vi "test Verify with Regex Scrubber.vi"(8 "error in":errorcluster, 11 "Test Case In":refnum<class "LUnit Extensions Tests.lvclass">) -> (0 "error out":errorcluster, 3 "Test Case Out":refnum<class "LUnit Extensions Tests.lvclass">)   [LabVIEW 2020, in "LUnit Extensions Tests.lvclass"]
uses:
  LUnit Extensions Tests.lvclass
  C:/Program Files/National Instruments/LabVIEW 2020/vi.lib/Astemes/LUnit/Test Case.lvclass
  Source/Approval Tests/Regex Scrubber/Regex Scrubber.lvclass
  <vilib>/Astemes/LUnit/Test Case.lvclass/Test Case.ctl
  240f995d-3744-484a-8956-6f48e6079b93.vi
  Source/Approval Tests/Regex Scrubber/Write Regex.vi
  Source/Approval Tests/Regex Scrubber/Write Replacement.vi
  240f995d-3744-484a-8956-6f48e6079b93.vi/1e051690-6811-4db0-8b8f-f6ad9423d026.vi
  <vilib>/Astemes/LUnit/Palette/Pass If.vi
  240f995d-3744-484a-8956-6f48e6079b93.vi/1e051690-6811-4db0-8b8f-f6ad9423d026.vi/93c5622b-9fb7-41e0-8c76-3fde37e94e34.vi
  <vilib>/Astemes/LUnit/Append Fail Result.vi
  <vilib>/Astemes/LUnit/Append Pass Result.vi
  240f995d-3744-484a-8956-6f48e6079b93.vi/1e051690-6811-4db0-8b8f-f6ad9423d026.vi/93c5622b-9fb7-41e0-8c76-3fde37e94e34.vi/daceb942-e4a5-48f9-868a-a7549e7f6e2f.vi
  Source/Approval Tests/Replace with Caller if Empty.vi
  Source/Approval Tests/conv EOL.vi
  Source/Approval Tests/Get Paths.vi
  <vilib>/Utility/libraryn.llb/Check if File or Folder Exists.vi
  Source/Approval Tests/Reporter/Reporter.lvclass
  Source/Approval Tests/Namer/Namer.lvclass
  Source/Approval Tests/Scrubber/Scrubber.lvclass
  LUnit Extensions Tests.lvclass/LUnit Extensions Tests.ctl
  Source/Approval Tests/Options.ctl
  Source/Approval Tests/Approval Tests.lvlib
  C:/Users/SAS/Desktop/ApprovalTests.LabVIEW/Source/Approval Tests/Regex Scrubber/Regex Scrubber.lvclass
  C:/Users/SAS/Desktop/ApprovalTests.LabVIEW/Source/Approval Tests/Scrubber/Scrubber.lvclass
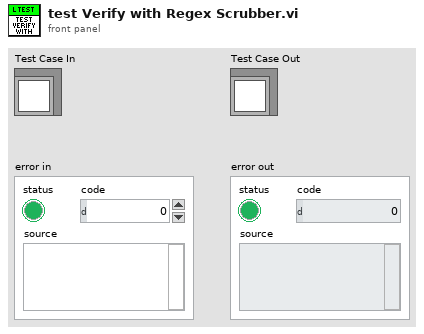
[diagram p1: front panel]
types:
  T1 = typedef "Approval Tests.lvlib/Options.ctl" = cluster{"Reporter":refnum<class "Reporter.lvclass">, "Extension(txt)":string, "Namer":refnum<class "Namer.lvclass">, "Scrubber":refnum<class "Scrubber.lvclass">}
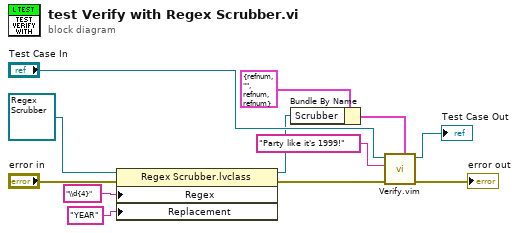
[diagram p0: block diagram]
diagram:
  n1 = property class="Regex Scrubber.lvclass"(reference=refnum<class "Regex Scrubber.lvclass"> refnum ("Approval Tests.lvlib:Regex Scrubber.lvclass"), error in="error in", "Regex"="\\d{4}", "Replacement"="YEAR") -> (reference out=w1:refnum<class "Regex Scrubber.lvclass">, error out=w5:errorcluster)
  n2 = Bundle By Name(cluster=T1 {"Reporter"=refnum, "Extension(txt)"="", "Namer"=refnum, "Scrubber"=refnum} ("Options"), "Scrubber"=w1) -> (w2:T1)
  n3 = call "Verify.vim"("Options"=w2, "error in"=w5, "Test Data"="Party like it's 1999!", "LUnit Test Case In"="Test Case In") -> ("error out"=→"error out":errorcluster, "LUnit Test Case Out"=→"Test Case Out":refnum<class "LUnit Extensions Tests.lvclass">)  [unwired: 6 in]
